vi "_TextTestResult.JUnitXML_Init.vi"(8 "error in (no error)":errorcluster, 10 "stream.Results":refnum<queue>, 11 "TestTestResult in":refnum<class "_TextTestResult.JUnitXML.lvclass">) -> (0 "error out":errorcluster, 3 "TestTestResult out":refnum<class "_TextTestResult.JUnitXML.lvclass">)   [LabVIEW 2011, in "_TextTestResult.JUnitXML.lvclass"]
uses:
  _TextTestResult.JUnitXML.lvclass
  _TextTestResult.JUnitXML.lvclass/_TextTestResult.JUnitXML.ctl
panel:
  # "JKI VI Tester for LabVIEW\nhttp://jkisoft.com/vi-tester\nCopyright (C) 2007-2009, JKI <info@jkisoft.com>\nALL RIGHTS RESERVED"
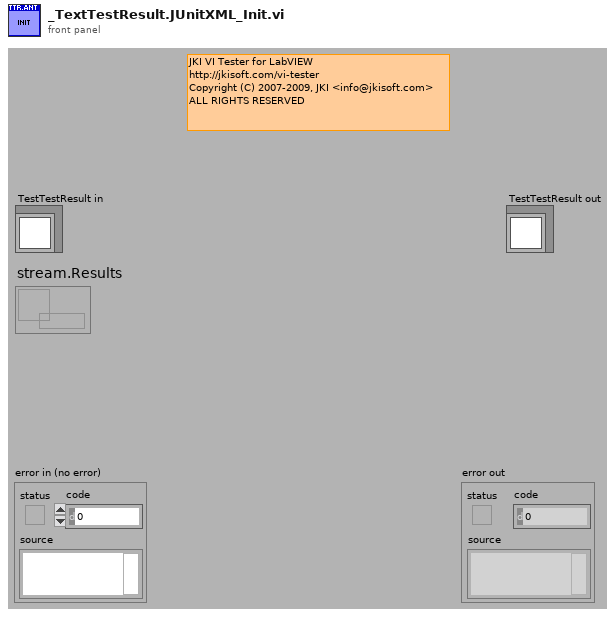
[diagram p1: front panel]
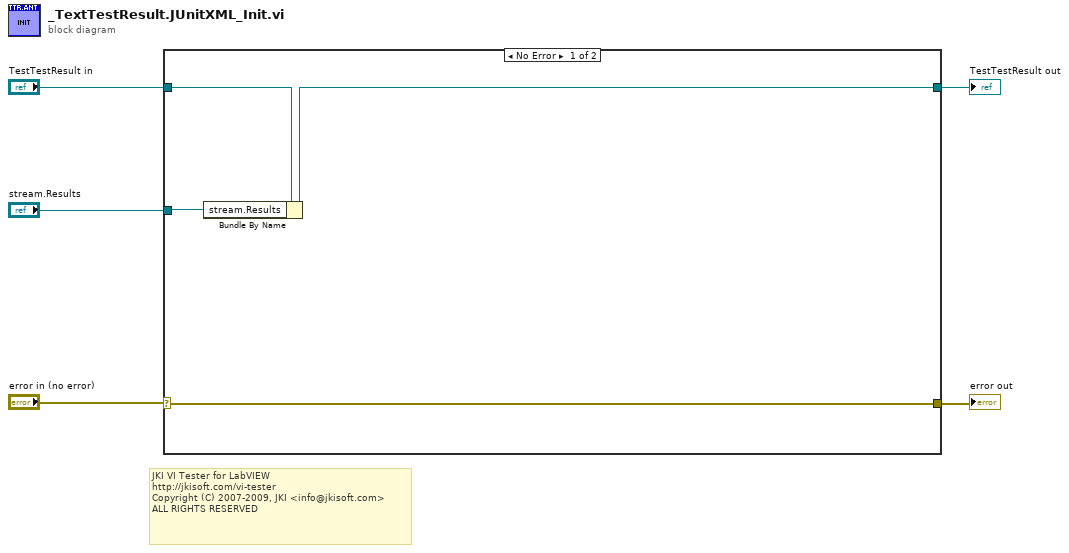
[diagram p0: block diagram]
diagram:
  # "JKI VI Tester for LabVIEW\nhttp://jkisoft.com/vi-tester\nCopyright (C) 2007-2009, JKI <info@jkisoft.com>\nALL RIGHTS RESERVED"
  n1 = case shown="No Error" "error in (no error)" {
    selector: "error in (no error)" -> [w7 w10]
    tunnel: "TestTestResult in" -> [w8 w11]
    tunnel: [w9 w11] -> w4
    tunnel: [w7 w10] -> w2
    tunnel: "stream.Results" -> [w6 _]
    frame No Error {
      n2 = Bundle By Name(cluster=w8, "stream.Results"=w6) -> (w9:refnum<class "_TextTestResult.JUnitXML.lvclass">)
    }
    frame Error {
    }
  }
  "TestTestResult out" <- w4
  "error out" <- w2
